vi "addFullyConnectedLayer.vi"(4 "NOUT":u32, 5 "ptr":i64, 6 "error in (no error)":errorcluster, 7 "path in":path) -> (0 "layers":u32, 1 "ptr out":i64, 2 "error out":errorcluster, 3 "path out":path)   [LabVIEW 2016, in "CNet.lvlib"]
uses:
  CNet.lvlib
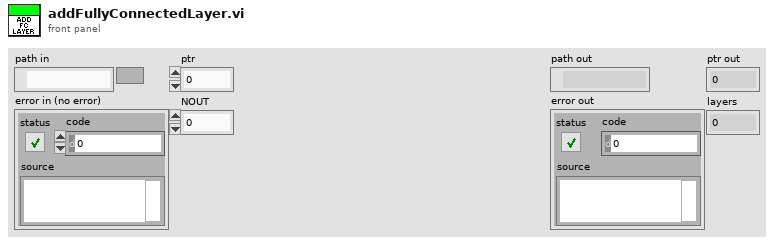
[diagram p1: front panel]
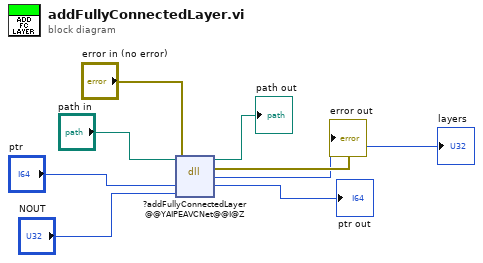
[diagram p0: block diagram]
diagram:
  n1 = dll-call lib="C:/Users/jg754/Documents/Visual Studio 2015/Projects/CLearn/x64/Debug/CLearn.dll" fn="?addFullyConnectedLayer@@YAIPEAVCNet@@I@Z"(path in="path in", error in="error in (no error)", "ptr"="ptr", "NOUT"="NOUT") -> (path out=→"path out":path, error out=→"error out":errorcluster, "layers"=→"layers":u32, "ptr"=→"ptr out":i64)  [unwired: 2 in]
